vi "TrajectoryConfig_Create.vi"(9 "MaxAcceleration":dbl, 11 "MaxVelocity":dbl) -> (3 "TRAJECTORY_CONFIG":T1 {"End Velocity" format="%20.4f"; "StartVelocity" format="%20.4f"; "Max Acceleration" format="%20.4f"; "MaxVelocity" format="%20.4f"})   [LabVIEW 2019, in "Trajectory_Library.lvlib"]
doc: "Constructs the trajectory configuration class.\n\nRepresents the configuration for generating a trajectory. This class stores the start velocity, end velocity, max velocity, max acceleration, custom constraints, and the reversed flag.\n \nThe cluster must be constructed with a max velocity and max acceleration. The other parameters (start velocity, end velocity, constraints, reversed) have been defaulted to reasonable values (0, 0, {}, false). These values can be changed via the setXXX methods.\n\nIt also contains the data for each contraint and a flag indicating if a particular constraint is active. As new constraints are added, this cluster will be modified to conain them.\n\nParameters:\n - maxVelocity - The max velocity for the trajectory. (Meters/Sec)\n - maxAcceleration - The max acceleration for the trajectory. (Meters/Sec^2)\n\nReturns:\n - TrajectoryConfig - TrajectoryConfig data structure"
uses:
  Trajectory_Library.lvlib
  TypeDef/TRAJ_CONFIG.ctl
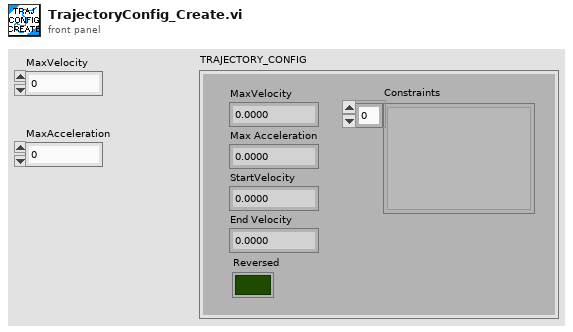
[diagram p1: front panel]
types:
  T1 = typedef "Trajectory_Library.lvlib/TRAJ_CONFIG.ctl" = cluster{"MaxVelocity":dbl, "Max Acceleration":dbl, "StartVelocity":dbl, "End Velocity":dbl, "Reversed":bool, "Constraints":variant[]}
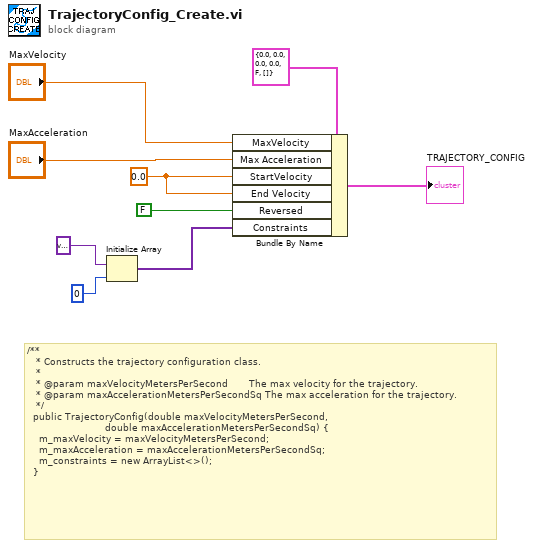
[diagram p0: block diagram]
diagram:
  w5 = 0.0 ("StartVelocity")
  # "/**\n   * Constructs the trajectory configuration class.\n   *\n   * @param maxVelocityMetersPerSecond       The max velocity for the trajectory.\n   * @param maxAccelerationMetersPerSecondSq The max acceleration for the trajectory.\n   */\n  public TrajectoryConfig(double maxVelocityMetersPerSecond,\n                          double maxAccelerationMetersPerSecondSq) {\n    m_maxVelocity = maxVelocityMetersPerSecond;\n    m_maxAcceleration = maxAccelerationMetersPerSecondSq;\n    m_constraints = new ArrayList<>();\n  }"
  n1 = Initialize Array(variant, 0 ("dimension size")) -> (w3:variant[])
  n2 = Bundle By Name(cluster=T1 {"MaxVelocity"=0.0, "Max Acceleration"=0.0, "StartVelocity"=0.0, "End Velocity"=0.0, "Reversed"=FALSE, "Constraints"=[]} ("TRAJECTORY_CONFIG"), "MaxVelocity"="MaxVelocity", "Max Acceleration"="MaxAcceleration", "StartVelocity"=w5, "End Velocity"=w5, "Reversed"=FALSE, "Constraints"=w3) -> (→"TRAJECTORY_CONFIG":T1)
